vi "LEDWithBOT_Main.vi"() -> ()   [LabVIEW 2014]
uses:
  TelegramBOT_class/SendMsgType.ctl
  TelegramBOT_class/KeyboardMarkup.ctl
  <vilib>/MakerHub/LINX/Public/Peripherals/Digital/Digital Write 1 Chan.vi
  <vilib>/MakerHub/LINX/Public/Peripherals/Digital/Digital Write N Chans.vi
  <vilib>/MakerHub/LINX/Private/Local IO/LinxDigitalWrite.vi
  <vilib>/MakerHub/LINX/Public/Utilities/Check Channel.vi
  <vilib>/MakerHub/LINX/Private/Local IO/Handle Errors.vi
  <vilib>/MakerHub/LINX/Public/Utilities/Open Local.vi
  <vilib>/MakerHub/LINX/Private/Utilties/Generate Error.vi
  TelegramBOT_class/TelegramBOT.lvclass
  <vilib>/MakerHub/LINX/LMH-LINX.lvlib
panel:
  out "text":string
  out "Msg":i32
  out "Connection":bool
  out "Error Out":errorcluster
  out "LED":bool
  in  "Stop":bool
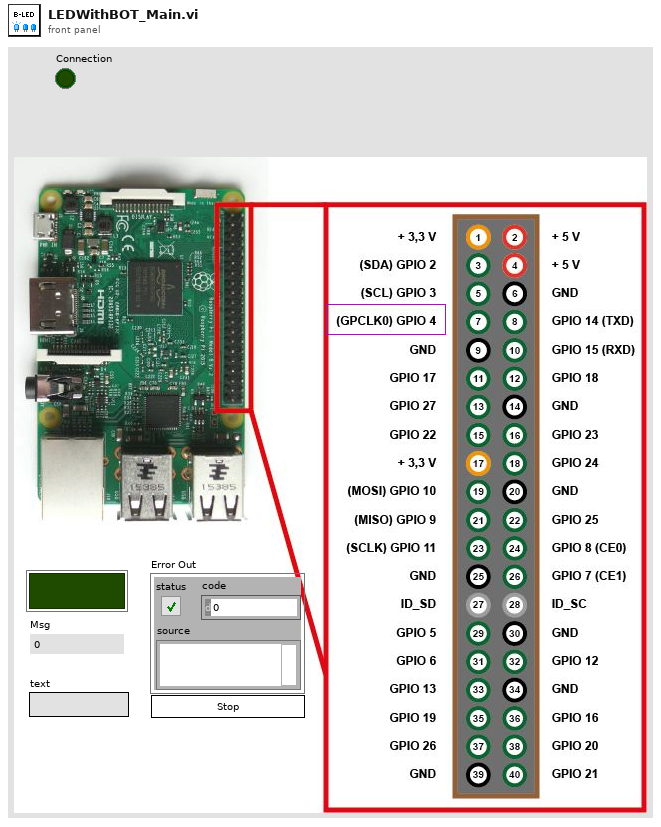
[diagram p1: front panel]
types:
  T1 = typedef "LMH-LINX.lvlib/LINX Ref.ctl" = cluster{"IO":T2, "Interface":T3, "LINX Device Config":T4}
  T2 = typedef "LMH-LINX.lvlib/Platform.ctl" = enum16{"Remote", "Local"}
  T3 = typedef "LMH-LINX.lvlib/Interface.ctl" = enum16{"Serial", "TCP"}
  T4 = typedef "LMH-LINX.lvlib/Device.lvlib/LINX Device Config.ctl" = cluster{"Interface":T3, "COM Port":refnum<visa-resource-name>, "TCP Configuration":T5, "Device Family":u8, "Device ID":u8, "Device Name":string, "TCP Ref":refnum<k5>, "Channels":T6}
  T5 = typedef "LMH-LINX.lvlib/Device.lvlib/TCP Config.ctl" = cluster{"IP Address":string, "Port":u16}
  T6 = typedef "LMH-LINX.lvlib/Channels.ctl" = cluster{"DI":u8[], "DO":u8[], "AI":u8[], "AO":u8[], "PWM":u8[], "QE":u8[], "UART":u8[], "I2C 2":u8[], "SPI":u8[], "CAN":u8[], "Servo":u8[], "AI Ref (V)":dbl, "AI Resolution (Bits)":u8, "AO Ref (V)":dbl, "AO Resolution (Bits)":u8}
  T7 = typedef "TelegramBOT.lvclass/KeyboardMarkup.ctl" = cluster{"keyboard":cluster{"text":string, "req_loc":bool}[][], "resize_keyboard":bool, "one_time_keyboard":bool, "selective":bool}
  T8 = typedef "TelegramBOT.lvclass/SendMsgType.ctl" = enum16{"Text", "ReplyKeyboardMarkup", "ReplyKeyboardRemove"}
  T9 = typedef "TelegramBOT.lvclass/MessageCluster.ctl" = cluster{"update_id":u32, "from":string, "text":string, "date":timestamp, "chat_id":i32, "type":string, "reply_to_message.text":string, "message_id":u32}
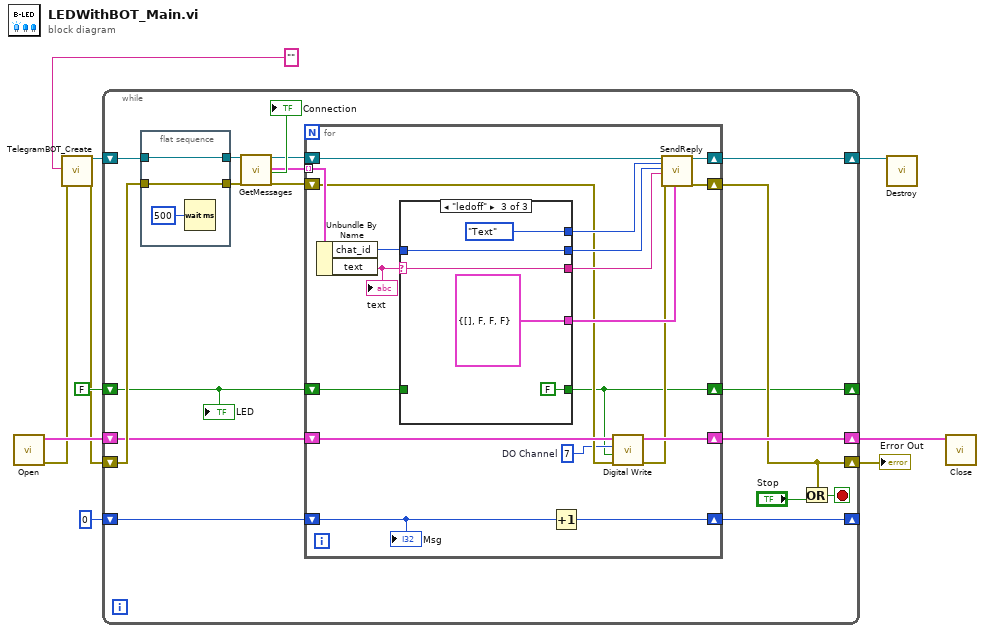
[diagram p0: block diagram]
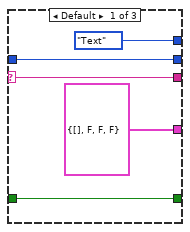
[diagram p2: hidden frame]
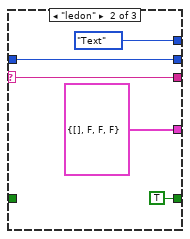
[diagram p3: hidden frame]
diagram:
  n1 = call-poly <vilib>:"Open.vi"() -> ("Error Out"=w4:errorcluster, "LINX Resource"=w10:T1)  [unwired: 9 in, 1 out]
  n2 = call "TelegramBOT_Create.vi"("BOTToken"="", "error in (no error)"=w4) -> ("reference out"=w6:refnum<class "TelegramBOT.lvclass">, "error out"=w3:errorcluster)  [unwired: 16 in]
  n3 = while {
    shift-right: [w16] -> w8
    shift-left: w10 -> [w17]
    shift-right: [w15] -> w7
    shift-left: w3 -> [w23]
    shift-right: [w13] -> _
    shift-left: FALSE -> [w14]
    shift-right: [w21] -> w2
    shift-left: w6 -> [w24]
    shift-right: [w11] -> _
    shift-left: 0 -> [w12]
    stop <- w27 stop-if-true
    n4 = flat-sequence {
      tunnel: [w65] -> w25
      tunnel: w24 -> [w65]
      tunnel: [w64] -> w26
      tunnel: w23 -> [w64]
      frame #0 {
        n5 = Wait (ms)(milliseconds to wait=u32 500) -> ()  [unwired: 1 out]
      }
    }
    n6 = call-dynamic "GetMessages.vi"("reference in"=w25, "error in (no error)"=w26) -> ("reference out"=w20:refnum<class "TelegramBOT.lvclass">, "Messages"=w19:T9[], "Connection"=→"Connection":bool, "error out"=w18:errorcluster)  [unwired: 13 in, 1 out]
    n7 = for {
      shift-right: [w43] -> w21
      shift-left: w20 -> [w44]
      shift-right: [w42] -> w15
      shift-left: w18 -> [w33]
      tunnel: w19 -> [w47] mode=indexing
      shift-right: [w36] -> w16
      shift-left: w17 -> [w34]
      shift-right: [w31] -> w13
      shift-left: w14 -> [w37]
      shift-right: [w29] -> w11
      shift-left: w12 -> [w30]
      w32 = u8 7  # DO Channel
      n8 = Unbundle By Name(w47) -> ("chat_id"=w45:i32, "text"=w46:string)
      "text" <- w46
      n9 = case shown="\"ledoff\"" w46 {
        selector: w46 -> [w52 w57 w62]
        tunnel: w45 -> [w51 w56 w61]
        tunnel: [w52 w57 w62] -> w41
        tunnel: [w51 w56 w61] -> w40
        tunnel: [SendMsgType."Text" ("MsgType") SendMsgType."Text" ("MsgType") SendMsgType."Text" ("MsgType")] -> w39
        tunnel: [T7 {"keyboard"=[], "resize_keyboard"=FALSE, "one_time_keyboard"=FALSE, "selective"=FALSE} ("ReplyKeyboardMarkup") T7 {"keyboard"=[], "resize_keyboard"=FALSE, "one_time_keyboard"=FALSE, "selective"=FALSE} ("ReplyKeyboardMarkup") T7 {"keyboard"=[], "resize_keyboard"=FALSE, "one_time_keyboard"=FALSE, "selective"=FALSE} ("ReplyKeyboardMarkup")] -> w38
        tunnel: w37 -> [w48 _ _]
        tunnel: [w48 TRUE FALSE] -> w31
        frame Default {
        }
        frame "ledon" {
        }
        frame "ledoff" {
        }
      }
      n10 = Increment(x=w30) -> (x+1=w29:i32)
      n11 = call-poly <vilib>:"Digital Write.vi"("Error In"=w33, "Output Value"=w31, "DO Channel"=w32, "LINX Resource"=w34) -> ("Error Out"=w35:errorcluster, "LINX Resource"=w36:T1)  [unwired: 6 in]
      n12 = call-dynamic "SendReply.vi"("reference in"=w44, "MsgType"=w39, "ChatId"=w40, "Text"=w41, "error in (no error)"=w35, "ReplyKeyboardMarkup"=w38) -> ("reference out"=w43:refnum<class "TelegramBOT.lvclass">, "error out"=w42:errorcluster)  [unwired: 12 in]
      "Msg" <- w30
    }
    n13 = Or(x=w15, y="Stop") -> (x .or. y?=w27:bool)
    "LED" <- w14
  }
  "Error Out" <- w7
  n14 = call-dynamic "Destroy.vi"("reference in"=w2) -> ()  [unwired: 17 in, 2 out]
  n15 = call <vilib>:"Close.vi"("LINX Resource"=w8) -> ()  [unwired: 10 in, 1 out]
